vi "canDataSort.vi"() -> ()   [LabVIEW 2023] (continued)
    3823  0CF102A7   00000004    8        30\t75\tE0\t2E\t80\tFF\tFF\tFD\r\n      3823  0CF101A7   00000004    8        68\t00\t97\tCC\t00\t19\t39\tD9\r\n      3822  1FFFFFFF   00000004    8        00\t20\tFF\tFF\tFF\tFF\tFF\tFF\r\n      3812  1FFFFFFF   00000004    8        00\t00\tFF\tFF\tFF\tFF\tFF\tFF\r\n      3803  0CF102A7   00000004    8        30\t75\tE0\t2E\t80\tFF\tFF\tFD\r\n      3844  0CF103A7   00000004    8        17\t1F\t08\t60\tB1\t1F\t08\t5E\r\n      3844  0CF102A7   00000004    8        30\t75\tE0\t2E\t80\tFF\tFF\tFD\r\n      3843  0C3C4D4A   00000004    8        BE\tFF\tFF\t7F\t18\tFF\tFF\t5E\r\n      3843  0CF101A7   00000004    8        68\t00\t97\tCC\t00\t19\t39\tDA\r\n      3842  18F120F0   00000004    8        2B\t75\t60\tB1\tB0\t01\tFF\tFF\r\n      3841  18F11FF0   00000004    8        FF\t3F\t90\t68\t88\t1B\t10\tEC\r\n      3832  1FFFFFFF   00000004    8        00\t00\tFF\tFF\tFF\tFF\tFF\tFF\r\n      3823  0CF102A7   00000004    8        30\t75\tE0\t2E\t80\tFF\tFF\tFD\r\n      3823  0CF101A7   00000004    8        68\t00\t97\tCC\t00\t19\t39\tD9\r\n      3822  1FFFFFFF   00000004    8        00\t20\tFF\tFF\tFF\tFF\tFF\tFF\r\n      3812  1FFFFFFF   00000004    8        00\t00\tFF\tFF\tFF\tFF\tFF\tFF\r\n      3845  0CF104A7   00000004    8        F0\t60\t22\tFC\tFF\tFF\tFF\t5E\r\n      3844  0CF103A7   00000004    8        17\t1F\t08\t60\tB1\t1F\t08\t5E\r\n      3844  0CF102A7   00000004    8        30\t75\tE0\t2E\t80\tFF\tFF\tFD\r\n      3843  0C3C4D4A   00000004    8        BE\tFF\tFF\t7F\t18\tFF\tFF\t5E\r\n      3843  0CF101A7   00000004    8        68\t00\t97\tCC\t00\t19\t39\tDA\r\n      3842  18F120F0   00000004    8        2B\t75\t60\tB1\tB0\t01\tFF\tFF\r\n      3841  18F11FF0   00000004    8        FF\t3F\t90\t68\t88\t1B\t10\tEC\r\n      3832  1FFFFFFF   00000004    8        00\t00\tFF\tFF\tFF\tFF\tFF\tFF\r\n      3823  0CF102A7   00000004    8        30\t75\tE0\t2E\t80\tFF\tFF\tFD\r\n      3823  0CF101A7   00000004    8        68\t00\t97\tCC\t00\t19\t39\tD9\r\n      3822  1FFFFFFF   00000004    8        00\t20\tFF\tFF\tFF\tFF\tFF\tFF\r\n      3845  18F106A7   00000004    8        00\tF7\tFF\tFF\tFF\tFF\tFF\tBD\r\n      3845  0CF104A7   00000004    8        F0\t60\t22\tFC\tFF\tFF\tFF\t5E\r\n      3844  0CF103A7   00000004    8        17\t1F\t08\t60\tB1\t1F\t08\t5E\r\n      3844  0CF102A7   00000004    8        30\t75\tE0\t2E\t80\tFF\tFF\tFD\r\n      3843  0C3C4D4A   00000004    8        BE\tFF\tFF\t7F\t18\tFF\tFF\t5E\r\n      3843  0CF101A7   00000004    8        68\t00\t97\tCC\t00\t19\t39\tDA\r\n      3842  18F120F0   00000004    8        2B\t75\t60\tB1\tB0\t01\tFF\tFF\r\n      3841  18F11FF0   00000004    8        FF\t3F\t90\t68\t88\t1B\t10\tEC\r\n      3832  1FFFFFFF   00000004    8        00\t00\tFF\tFF\tFF\tFF\tFF\tFF\r\n      3823  0CF102A7   00000004    8        30\t75\tE0\t2E\t80\tFF\tFF\tFD\r\n      3823  0CF101A7   00000004    8        68\t00\t97\tCC\t00\t19\t39\tD9\r\n      3846  18F121F0   00000004    8        09\t33\t00\t00\tFF\tFF\tB0\t01\r\n      3845  18F106A7   00000004    8        00\tF7\tFF\tFF\tFF\tFF\tFF\tBD\r\n      3845  0CF104A7   00000004    8        F0\t60\t22\tFC\tFF\tFF\tFF\t5E\r\n      3844  0CF103A7   00000004    8        17\t1F\t08\t60\tB1\t1F\t08\t5E\r\n      3844  0CF102A7   00000004    8        30\t75\tE0\t2E\t80\tFF\tFF\tFD\r\n      3843  0C3C4D4A   00000004    8        BE\tFF\tFF\t7F\t18\tFF\tFF\t5E\r\n      3843  0CF101A7   00000004    8        68\t00\t97\tCC\t00\t19\t39\tDA\r\n      3842  18F120F0   00000004    8        2B\t75\t60\tB1\tB0\t01\tFF\tFF\r\n      3841  18F11FF0   00000004    8        FF\t3F\t90\t68\t88\t1B\t10\tEC\r\n      3832  1FFFFFFF   00000004    8        00\t00\tFF\tFF\tFF\tFF\tFF\tFF\r\n      3823  0CF102A7   00000004    8        30\t75\tE0\t2E\t80\tFF\tFF\tFD\r\n      3847  1FFFFFFF   00000004    8        00\t00\tFF\tFF\tFF\tFF\tFF\tFF\r\n      3846  18F121F0   00000004    8        09\t33\t00\t00\tFF\tFF\tB0\t01\r\n      3845  18F106A7   00000004    8        00\tF7\tFF\tFF\tFF\tFF\tFF\tBD\r\n      3845  0CF104A7   00000004    8        F0\t60\t22\tFC\tFF\tFF\tFF\t5E\r\n      3844  0CF103A7   00000004    8        17\t1F\t08\t60\tB1\t1F\t08\t5E\r\n      3844  0CF102A7   00000004    8        30\t75\tE0\t2E\t80\tFF\tFF\tFD\r\n      3843  0C3C4D4A   00000004    8        BE\tFF\tFF\t7F\t18\tFF\tFF\t5E\r\n      3843  0CF101A7   00000004    8        68\t00\t97\tCC\t00\t19\t39\tDA\r\n      3842  18F120F0   00000004    8        2B\t75\t60\tB1\tB0\t01\tFF\tFF\r\n      3841  18F11FF0   00000004    8        FF\t3F\t90\t68\t88\t1B\t10\tEC\r\n      3832  1FFFFFFF   00000004    8        00\t00\tFF\tFF\tFF\tFF\tFF\tFF\r\n      3852  1FFFFFFF   00000004    8        00\t00\tFF\tFF\tFF\tFF\tFF\tFF\r\n      3847  1FFFFFFF   00000004    8        00\t00\tFF\tFF\tFF\tFF\tFF\tFF\r\n      3846  18F121F0   00000004    8        09\t33\t00\t00\tFF\tFF\tB0\t01\r\n      3845  18F106A7   00000004    8        00\tF7\tFF\tFF\tFF\tFF\tFF\tBD\r\n      3845  0CF104A7   00000004    8        F0\t60\t22\tFC\tFF\tFF\tFF\t5E\r\n      3844  0CF103A7   00000004    8        17\t1F\t08\t60\tB1\t1F\t08\t5E\r\n      3844  0CF102A7   00000004    8        30\t75\tE0\t2E\t80\tFF\tFF\tFD\r\n      3843  0C3C4D4A   00000004    8        BE\tFF\tFF\t7F\t18\tFF\tFF\t5E\r\n      3843  0CF101A7   00000004    8        68\t00\t97\tCC\t00\t19\t39\tDA\r\n      3842  18F120F0   00000004    8        2B\t75\t60\tB1\tB0\t01\tFF\tFF\r\n      3841  18F11FF0   00000004    8        FF\t3F\t90\t68\t88\t1B\t10\tEC\r\n      3862  1FFFFFFF   00000004    8        00\t00\tFF\tFF\tFF\tFF\tFF\tFF\r\n      3852  1FFFFFFF   00000004    8        00\t00\tFF\tFF\tFF\tFF\tFF\tFF\r\n      3847  1FFFFFFF   00000004    8        00\t00\tFF\tFF\tFF\tFF\tFF\tFF\r\n      3846  18F121F0   00000004    8        09\t33\t00\t00\tFF\tFF\tB0\t01\r\n      3845  18F106A7   00000004    8        00\tF7\tFF\tFF\tFF\tFF\tFF\tBD\r\n      3845  0CF104A7   00000004    8        F0\t60\t22\tFC\tFF\tFF\tFF\t5E\r\n      3844  0CF103A7   00000004    8        17\t1F\t08\t60\tB1\t1F\t08\t5E\r\n      3844  0CF102A7   00000004    8        30\t75\tE0\t2E\t80\tFF\tFF\tFD\r\n      3843  0C3C4D4A   00000004    8        BE\tFF\tFF\t7F\t18\tFF\tFF\t5E\r\n      3843  0CF101A7   00000004    8        68\t00\t97\tCC\t00\t19\t39\tDA\r\n      3842  18F120F0   00000004    8        2B\t75\t60\tB1\tB0\t01\tFF\tFF\r\n      3863  0CF101A7   00000004    8        68\t00\t97\tCC\t00\t19\t39\tDB\r\n      3862  1FFFFFFF   00000004    8        00\t00\tFF\tFF\tFF\tFF\tFF\tFF\r\n      3852  1FFFFFFF   00000004    8        00\t00\tFF\tFF\tFF\tFF\tFF\tFF\r\n      3847  1FFFFFFF   00000004    8        00\t00\tFF\tFF\tFF\tFF\tFF\tFF\r\n      3846  18F121F0   00000004    8        09\t33\t00\t00\tFF\tFF\tB0\t01\r\n      3845  18F106A7   00000004    8        00\tF7\tFF\tFF\tFF\tFF\tFF\tBD\r\n      3845  0CF104A7   00000004    8        F0\t60\t22\tFC\tFF\tFF\tFF\t5E\r\n      3844  0CF103A7   00000004    8        17\t1F\t08\t60\tB1\t1F\t08\t5E\r\n      3844  0CF102A7   00000004    8        30\t75\tE0\t2E\t80\tFF\tFF\tFD\r\n      3843  0C3C4D4A   00000004    8        BE\tFF\tFF\t7F\t18\tFF\tFF\t5E\r\n      3843  0CF101A7   00000004    8        68\t00\t97\tCC\t00\t19\t39\tDA\r\n      3863  0CF102A7   00000004    8        30\t75\tE0\t2E\t80\tFF\tFF\tFD\r\n      3863  0CF101A7   00000004    8        68\t00\t97\tCC\t00\t19\t39\tDB\r\n      3862  1FFFFFFF   00000004    8        00\t00\tFF\tFF\tFF\tFF\tFF\tFF\r\n      3852  1FFFFFFF   00000004    8        00\t00\tFF\tFF\tFF\tFF\tFF\tFF\r\n      3847  1FFFFFFF   00000004    8        00\t00\tFF\tFF\tFF\tFF\tFF\tFF\r\n      3846  18F121F0   00000004    8        09\t33\t00\t00\tFF\tFF\tB0\t01\r\n      3845  18F106A7   00000004    8        00\tF7\tFF\tFF\tFF\tFF\tFF\tBD\r\n      3845  0CF104A7   00000004    8        F0\t60\t22\tFC\tFF\tFF\tFF\t5E\r\n      3844  0CF103A7   00000004    8        17\t1F\t08\t60\tB1\t1F\t08\t5E\r\n      3844  0CF102A7   00000004    8        30\t75\tE0\t2E\t80\tFF\tFF\tFD\r\n      3843  0C3C4D4A   00000004    8        BE\tFF\tFF\t7F\t18\tFF\tFF\t5E\r\n      3872  1FFFFFFF   00000004    8        00\t00\tFF\tFF\tFF\tFF\tFF\tFF\r\n      3863  0CF102A7   00000004    8        30\t75\tE0\t2E\t80\tFF\tFF\tFD\r\n      3863  0CF101A7   00000004    8        68\t00\t97\tCC\t00\t19\t39\tDB\r\n      3862  1FFFFFFF   00000004    8        00\t00\tFF\tFF\tFF\tFF\tFF\tFF\r\n      3852  1FFFFFFF   00000004    8        00\t00\tFF\tFF\tFF\tFF\tFF\tFF\r\n      3847  1FFFFFFF   00000004    8        00\t00\tFF\tFF\tFF\tFF\tFF\tFF\r\n      3846  18F121F0   00000004    8        09\t33\t00\t00\tFF\tFF\tB0\t01\r\n      3845  18F106A7   00000004    8        00\tF7\tFF\tFF\tFF\tFF\tFF\tBD\r\n      3845  0CF104A7   00000004    8        F0\t60\t22\tFC\tFF\tFF\tFF\t5E\r\n      3844  0CF103A7   00000004    8        17\t1F\t08\t60\tB1\t1F\t08\t5E\r\n      3844  0CF102A7   00000004    8        30\t75\tE0\t2E\t80\tFF\tFF\tFD\r\n      3882  1FFFFFFF   00000004    8        00\t00\tFF\tFF\tFF\tFF\tFF\tFF\r\n      3872  1FFFFFFF   00000004    8        00\t00\tFF\tFF\tFF\tFF\tFF\tFF\r\n      3863  0CF102A7   00000004    8        30\t75\tE0\t2E\t80\tFF\tFF\tFD\r\n      3863  0CF101A7   00000004    8        68\t00\t97\tCC\t00\t19\t39\tDB\r\n      3862  1FFFFFFF   00000004    8        00\t00\tFF\tFF\tFF\tFF\tFF\tFF\r\n      3852  1FFFFFFF   00000004    8        00\t00\tFF\tFF\tFF\tFF\tFF\tFF\r\n      3847  1FFFFFFF   00000004    8        00\t00\tFF\tFF\tFF\tFF\tFF\tFF\r\n      3846  18F121F0   00000004    8        09\t33\t00\t00\tFF\tFF\tB0\t01\r\n      3845  18F106A7   00000004    8        00\tF7\tFF\tFF\tFF\tFF\tFF\tBD\r\n      3845  0CF104A7   00000004    8        F0\t60\t22\tFC\tFF\tFF\tFF\t5E\r\n      3844  0CF103A7   00000004    8        17\t1F\t08\t60\tB1\t1F\t08\t5E\r\n      3883  0CF101A7   00000004    8        68\t00\t97\tCC\t00\t19\t39\tDC\r\n      3882  1FFFFFFF   00000004    8        00\t00\tFF\tFF\tFF\tFF\tFF\tFF\r\n      3872  1FFFFFFF   00000004    8        00\t00\tFF\tFF\tFF\tFF\tFF\tFF\r\n      3863  0CF102A7   00000004    8        30\t75\tE0\t2E\t80\tFF\tFF\tFD\r\n      3863  0CF101A7   00000004    8        68\t00\t97\tCC\t00\t19\t39\tDB\r\n      3862  1FFFFFFF   00000004    8        00\t00\tFF\tFF\tFF\tFF\tFF\tFF\r\n      3852  1FFFFFFF   00000004    8        00\t00\tFF\tFF\tFF\tFF\tFF\tFF\r\n      3847  1FFFFFFF   00000004    8        00\t00\tFF\tFF\tFF\tFF\tFF\tFF\r\n      3846  18F121F0   00000004    8        09\t33\t00\t00\tFF\tFF\tB0\t01\r\n      3845  18F106A7   00000004    8        00\tF7\tFF\tFF\tFF\tFF\tFF\tBD\r\n      3845  0CF104A7   00000004    8        F0\t60\t22\tFC\tFF\tFF\tFF\t5E\r\n      3883  0CF102A7   00000004    8        30\t75\tE0\t2E\t80\tFF\tFF\tFD\r\n      3883  0CF101A7   00000004    8        68\t00\t97\tCC\t00\t19\t39\tDC\r\n      3882  1FFFFFFF   00000004    8        00\t00\tFF\tFF\tFF\tFF\tFF\tFF\r\n      3872  1FFFFFFF   00000004    8        00\t00\tFF\tFF\tFF\tFF\tFF\tFF\r\n      3863  0CF102A7   00000004    8        30\t75\tE0\t2E\t80\tFF\tFF\tFD\r\n      3863  0CF101A7   00000004    8        68\t00\t97\tCC\t00\t19\t39\tDB\r\n      3862  1FFFFFFF   00000004    8        00\t00\tFF\tFF\tFF\tFF\tFF\tFF\r\n      3852  1FFFFFFF   00000004    8        00\t00\tFF\tFF\tFF\tFF\tFF\tFF\r\n      3847  1FFFFFFF   00000004    8        00\t00\tFF\tFF\tFF\tFF\tFF\tFF\r\n      3846  18F121F0   00000004    8        09\t33\t00\t00\tFF\tFF\tB0\t01\r\n      3845  18F106A7   00000004    8        00\tF7\tFF\tFF\tFF\tFF\tFF\tBD\r\n      3892  1FFFFFFF   00000004    8        00\t00\tFF\tFF\tFF\tFF\tFF\tFF\r\n      3883  0CF102A7   00000004    8        30\t75\tE0\t2E\t80\tFF\tFF\tFD\r\n      3883  0CF101A7   00000004    8        68\t00\t97\tCC\t00\t19\t39\tDC\r\n      3882  1FFFFFFF   00000004    8        00\t00\tFF\tFF\tFF\tFF\tFF\tFF\r\n      3872  1FFFFFFF   00000004    8        00\t00\tFF\tFF\tFF\tFF\tFF\tFF\r\n      3863  0CF102A7   00000004    8        30\t75\tE0\t2E\t80\tFF\tFF\tFD\r\n      3863  0CF101A7   00000004    8        68\t00\t97\tCC\t00\t19\t39\tDB\r\n      3862  1FFFFFFF   00000004    8        00\t00\tFF\tFF\tFF\tFF\tFF\tFF\r\n      3852  1FFFFFFF   00000004    8        00\t00\tFF\tFF\tFF\tFF\tFF\tFF\r\n      3847  1FFFFFFF   00000004    8        00\t00\tFF\tFF\tFF\tFF\tFF\tFF\r\n      3846  18F121F0   00000004    8        09\t33\t00\t00\tFF\tFF\tB0\t01\r\n      3893  18F106A7   00000004    8        00\tF7\tFF\tFF\tFF\tFF\tFF\tBE\r\n      3892  1FFFFFFF   00000004    8        00\t00\tFF\tFF\tFF\tFF\tFF\tFF\r\n      3883  0CF102A7   00000004    8        30\t75\tE0\t2E\t80\tFF\tFF\tFD\r\n      3883  0CF101A7   00000004    8        68\t00\t97\tCC\t00\t19\t39\tDC\r\n      3882  1FFFFFFF   00000004    8        00\t00\tFF\tFF\tFF\tFF\tFF\tFF\r\n      3872  1FFFFFFF   00000004    8        00\t00\tFF\tFF\tFF\tFF\tFF\tFF\r\n      3863  0CF102A7   00000004    8        30\t75\tE0\t2E\t80\tFF\tFF\tFD\r\n      3863  0CF101A7   00000004    8        68\t00\t97\tCC\t00\t19\t39\tDB\r\n      3862  1FFFFFFF   00000004    8        00\t00\tFF\tFF\tFF\tFF\tFF\tFF\r\n      3852  1FFFFFFF   00000004    8        00\t00\tFF\tFF\tFF\tFF\tFF\tFF\r\n      3847  1FFFFFFF   00000004    8        00\t00\tFF\tFF\tFF\tFF\tFF\tFF\r\n      3902  1FFFFFFF   00000004    8        00\t20\tFF\tFF\tFF\tFF\tFF\tFF\r\n      3893  18F106A7   00000004    8        00\tF7\tFF\tFF\tFF\tFF\tFF\tBE\r\n      3892  1FFFFFFF   00000004    8        00\t00\tFF\tFF\tFF\tFF\tFF\tFF\r\n      3883  0CF102A7   00000004    8        30\t75\tE0\t2E\t80\tFF\tFF\tFD\r\n      3883  0CF101A7   00000004    8        68\t00\t97\tCC\t00\t19\t39\tDC\r\n      3882  1FFFFFFF   00000004    8        00\t00\tFF\tFF\tFF\tFF\tFF\tFF\r\n      3872  1FFFFFFF   00000004    8        00\t00\tFF\tFF\tFF\tFF\tFF\tFF\r\n      3863  0CF102A7   00000004    8        30\t75\tE0\t2E\t80\tFF\tFF\tFD\r\n      3863  0CF101A7   00000004    8        68\t00\t97\tCC\t00\t19\t39\tDB\r\n      3862  1FFFFFFF   00000004    8        00\t00\tFF\tFF\tFF\tFF\tFF\tFF\r\n      3852  1FFFFFFF   00000004    8        00\t00\tFF\tFF\tFF\tFF\tFF\tFF\r\n      3902  0CF101A7   00000004    8        68\t00\t97\tCC\t00\t19\t39\tDD\r\n      3902  1FFFFFFF   00000004    8        00\t20\tFF\tFF\tFF\tFF\tFF\tFF\r\n      3893  18F106A7   00000004    8        00\tF7\tFF\tFF\tFF\tFF\tFF\tBE\r\n      3892  1FFFFFFF   00000004    8        00\t00\tFF\tFF\tFF\tFF\tFF\tFF\r\n      3883  0CF102A7   00000004    8        30\t75\tE0\t2E\t80\tFF\tFF\tFD\r\n      3883  0CF101A7   00000004    8        68\t00\t97\tCC\t00\t19\t39\tDC\r\n      3882  1FFFFFFF   00000004    8        00\t00\tFF\tFF\tFF\tFF\tFF\tFF\r\n      3872  1FFFFFFF   00000004    8        00\t00\tFF\tFF\tFF\tFF\tFF\tFF\r\n      3863  0CF102A7   00000004    8        30\t75\tE0\t2E\t80\tFF\tFF\tFD\r\n      3863  0CF101A7   00000004    8        68\t00\t97\tCC\t00\t19\t39\tDB\r\n      3862  1FFFFFFF   00000004    8        00\t00\tFF\tFF\tFF\tFF\tFF\tFF\r\n      3903  0CF102A7   00000004    8        30\t75\tE0\t2E\t80\tFF\tFF\tFD\r\n      3902  0CF101A7   00000004    8        68\t00\t97\tCC\t00\t19\t39\tDD\r\n      3902  1FFFFFFF   00000004    8        00\t20\tFF\tFF\tFF\tFF\tFF\tFF\r\n      3893  18F106A7   00000004    8        00\tF7\tFF\tFF\tFF\tFF\tFF\tBE\r\n      3892  1FFFFFFF   00000004    8        00\t00\tFF\tFF\tFF\tFF\tFF\tFF\r\n      3883  0CF102A7   00000004    8        30\t75\tE0\t2E\t80\tFF\tFF\tFD\r\n      3883  0CF101A7   00000004    8        68\t00\t97\tCC\t00\t19\t39\tDC\r\n      3882  1FFFFFFF   00000004    8        00\t00\tFF\tFF\tFF\tFF\tFF\tFF\r\n      3872  1FFFFFFF   00000004    8        00\t00\tFF\tFF\tFF\tFF\tFF\tFF\r\n      3863  0CF102A7   00000004    8        30\t75\tE0\t2E\t80\tFF\tFF\tFD\r\n      3863  0CF101A7   00000004    8        68\t00\t97\tCC\t00\t19\t39\tDB\r\n      3912  1FFFFFFF   00000004    8        00\t00\tFF\tFF\tFF\tFF\tFF\tFF\r\n      3903  0CF102A7   00000004    8        30\t75\tE0\t2E\t80\tFF\tFF\tFD\r\n      3902  0CF101A7   00000004    8        68\t00\t97\tCC\t00\t19\t39\tDD\r\n      3902  1FFFFFFF   00000004    8        00\t20\tFF\tFF\tFF\tFF\tFF\tFF\r\n      3893  18F106A7   00000004    8        00\tF7\tFF\tFF\tFF\tFF\tFF\tBE\r\n      3892  1FFFFFFF   00000004    8        00\t00\tFF\tFF\tFF\tFF\tFF\tFF\r\n      3883  0CF102A7   00000004    8        30\t75\tE0\t2E\t80\tFF\tFF\tFD\r\n      3883  0CF101A7   00000004    8        68\t00\t97\tCC\t00\t19\t39\tDC\r\n      3882  1FFFFFFF   00000004    8        00\t00\tFF\tFF\tFF\tFF\tFF\tFF\r\n      3872  1FFFFFFF   00000004    8        00\t00\tFF\tFF\tFF\tFF\tFF\tFF\r\n      3863  0CF102A7   00000004    8        30\t75\tE0\t2E\t80\tFF\tFF\tFD\r\n      3922  1FFFFFFF   00000004    8        00\t00\tFF\tFF\tFF\tFF\tFF\tFF\r\n      3912  1FFFFFFF   00000004    8        00\t00\tFF\tFF\tFF\tFF\tFF\tFF\r\n      3903  0CF102A7   00000004    8        30\t75\tE0\t2E\t80\tFF\tFF\tFD\r\n      3902  0CF101A7   00000004    8        68\t00\t97\tCC\t00\t19\t39\tDD\r\n      3902  1FFFFFFF   00000004    8        00\t20\tFF\tFF\tFF\tFF\tFF\tFF\r\n      3893  18F106A7   00000004    8        00\tF7\tFF\tFF\tFF\tFF\tFF\tBE\r\n      3892  1FFFFFFF   00000004    8        00\t00\tFF\tFF\tFF\tFF\tFF\tFF\r\n      3883  0CF102A7   00000004    8        30\t75\tE0\t2E\t80\tFF\tFF\tFD\r\n      3883  0CF101A7   00000004    8        68\t00\t97\tCC\t00\t19\t39\tDC\r\n      3882  1FFFFFFF   00000004    8        00\t00\tFF\tFF\tFF\tFF\tFF\tFF\r\n      3872  1FFFFFFF   00000004    8        00\t00\tFF\tFF\tFF\tFF\tFF\tFF\r\n      3923  0CF101A7   00000004    8        68\t00\t97\tCC\t00\t19\t39\tDE\r\n      3922  1FFFFFFF   00000004    8        00\t00\tFF\tFF\tFF\tFF\tFF\tFF\r\n      3912  1FFFFFFF   00000004    8        00\t00\tFF\tFF\tFF\tFF\tFF\tFF\r\n      3903  0CF102A7   00000004    8        30\t75\tE0\t2E\t80\tFF\tFF\tFD\r\n      3902  0CF101A7   00000004    8        68\t00\t97\tCC\t00\t19\t39\tDD\r\n      3902  1FFFFFFF   00000004    8        00\t20\tFF\tFF\tFF\tFF\tFF\tFF\r\n      3893  18F106A7   00000004    8        00\tF7\tFF\tFF\tFF\tFF\tFF\tBE\r\n      3892  1FFFFFFF   00000004    8        00\t00\tFF\tFF\tFF\tFF\tFF\tFF\r\n      3883  0CF102A7   00000004    8        30\t75\tE0\t2E\t80\tFF\tFF\tFD\r\n      3883  0CF101A7   00000004    8        68\t00\t97\tCC\t00\t19\t39\tDC\r\n      3882  1FFFFFFF   00000004    8        00\t00\tFF\tFF\tFF\tFF\tFF\tFF\r\n      3923  0CF102A7   00000004    8        30\t75\tE0\t2E\t80\tFF\tFF\tFD\r\n      3923  0CF101A7   00000004    8        68\t00\t97\tCC\t00\t19\t39\tDE\r\n      3922  1FFFFFFF   00000004    8        00\t00\tFF\tFF\tFF\tFF\tFF\tFF\r\n      3912  1FFFFFFF   00000004    8        00\t00\tFF\tFF\tFF\tFF\tFF\tFF\r\n      3903  0CF102A7   00000004    8        30\t75\tE0\t2E\t80\tFF\tFF\tFD\r\n      3902  0CF101A7   00000004    8        68\t00\t97\tCC\t00\t19\t39\tDD\r\n      3902  1FFFFFFF   00000004    8        00\t20\tFF\tFF\tFF\tFF\tFF\tFF\r\n      3893  18F106A7   00000004    8        00\tF7\tFF\tFF\tFF\tFF\tFF\tBE\r\n      3892  1FFFFFFF   00000004    8        00\t00\tFF\tFF\tFF\tFF\tFF\tFF\r\n      3883  0CF102A7   00000004    8        30\t75\tE0\t2E\t80\tFF\tFF\tFD\r\n      3883  0CF101A7   00000004    8        68\t00\t97\tCC\t00\t19\t39\tDC\r\n      3932  1FFFFFFF   00000004    8        00\t00\tFF\tFF\tFF\tFF\tFF\tFF\r\n      3923  0CF102A7   00000004    8        30\t75\tE0\t2E\t80\tFF\tFF\tFD\r\n      3923  0CF101A7   00000004    8        68\t00\t97\tCC\t00\t19\t39\tDE\r\n      3922  1FFFFFFF   00000004    8        00\t00\tFF\tFF\tFF\tFF\tFF\tFF\r\n      3912  1FFFFFFF   00000004    8        00\t00\tFF\tFF\tFF\tFF\tFF\tFF\r\n      3903  0CF102A7   00000004    8        30\t75\tE0\t2E\t80\tFF\tFF\tFD\r\n      3902  0CF101A7   00000004    8        68\t00\t97\tCC\t00\t19\t39\tDD\r\n      3902  1FFFFFFF   00000004    8        00\t20\tFF\tFF\tFF\tFF\tFF\tFF\r\n      3893  18F106A7   00000004    8        00\tF7\tFF\tFF\tFF\tFF\tFF\tBE\r\n      3892  1FFFFFFF   00000004    8        00\t00\tFF\tFF\tFF\tFF\tFF\tFF\r\n      3883  0CF102A7   00000004    8        30\t75\tE0\t2E\t80\tFF\tFF\tFD\r\n      3941  18F11FF0   00000004    8        FF\t3F\t90\t68\t88\t1B\t10\tFC\r\n      3932  1FFFFFFF   00000004    8        00\t00\tFF\tFF\tFF\tFF\tFF\tFF\r\n      3923  0CF102A7   00000004    8        30\t75\tE0\t2E\t80\tFF\tFF\tFD\r\n      3923  0CF101A7   00000004    8        68\t00\t97\tCC\t00\t19\t39\tDE\r\n      3922  1FFFFFFF   00000004    8        00\t00\tFF\tFF\tFF\tFF\tFF\tFF\r\n      3912  1FFFFFFF   00000004    8        00\t00\tFF\tFF\tFF\tFF\tFF\tFF\r\n      3903  0CF102A7   00000004    8        30\t75\tE0\t2E\t80\tFF\tFF\tFD\r\n      3902  0CF101A7   00000004    8        68\t00\t97\tCC\t00\t19\t39\tDD\r\n      3902  1FFFFFFF   00000004    8        00\t20\tFF\tFF\tFF\tFF\tFF\tFF\r\n      3893  18F106A7   00000004    8        00\tF7\tFF\tFF\tFF\tFF\tFF\tBE\r\n      3892  1FFFFFFF   00000004    8        00\t00\tFF\tFF\tFF\tFF\tFF\tFF\r\n      3942  18F120F0   00000004    8        2B\t75\t60\tB1\tB0\t01\tFF\tFF\r\n      3941  18F11FF0   00000004    8        FF\t3F\t90\t68\t88\t1B\t10\tFC\r\n      3932  1FFFFFFF   00000004    8        00\t00\tFF\tFF\tFF\tFF\tFF\tFF\r\n      3923  0CF102A7   00000004    8        30\t75\tE0\t2E\t80\tFF\tFF\tFD\r\n      3923  0CF101A7   00000004    8        68\t00\t97\tCC\t00\t19\t39\tDE\r\n      3922  1FFFFFFF   00000004    8        00\t00\tFF\tFF\tFF\tFF\tFF\tFF\r\n      3912  1FFFFFFF   00000004    8        00\t00\tFF\tFF\tFF\tFF\tFF\tFF\r\n      3903  0CF102A7   00000004    8        30\t75\tE0\t2E\t80\tFF\tFF\tFD\r\n      3902  0CF101A7   00000004    8        68\t00\t97\tCC\t00\t19\t39\tDD\r\n      3902  1FFFFFFF   00000004    8        00\t20\tFF\tFF\tFF\tFF\tFF\tFF\r\n      3893  18F106A7   00000004    8        00\tF7\tFF\tFF\tFF\tFF\tFF\tBE\r\n      3943  0CF101A7   00000004    8        68\t00\t97\tCC\t00\t19\t39\tDF\r\n      3942  18F120F0   00000004    8        2B\t75\t60\tB1\tB0\t01\tFF\tFF\r\n      3941  18F11FF0   00000004    8        FF\t3F\t90\t68\t88\t1B\t10\tFC\r\n      3932  1FFFFFFF   00000004    8        00\t00\tFF\tFF\tFF\tFF\tFF\tFF\r\n      3923  0CF102A7   00000004    8        30\t75\tE0\t2E\t80\tFF\tFF\tFD\r\n      3923  0CF101A7   00000004    8        68\t00\t97\tCC\t00\t19\t39\tDE\r\n      3922  1FFFFFFF   00000004    8        00\t00\tFF\tFF\tFF\tFF\tFF\tFF\r\n      3912  1FFFFFFF   00000004    8        00\t00\tFF\tFF\tFF\tFF\tFF\tFF\r\n      3903  0CF102A7   00000004    8        30\t75\tE0\t2E\t80\tFF\tFF\tFD\r\n      3902  0CF101A7   00000004    8        68\t00\t97\tCC\t00\t19\t39\tDD\r\n      3902  1FFFFFFF   00000004    8        00\t20\tFF\tFF\tFF\tFF\tFF\tFF\r\n      3943  0C3C4D4A   00000004    8        BE\tFF\tFF\t7F\t18\tFF\tFF\t5F\r\n      3943  0CF101A7   00000004    8        68\t00\t97\tCC\t00\t19\t39\tDF\r\n      3942  18F120F0   00000004    8        2B\t75\t60\tB1\tB0\t01\tFF\tFF\r\n      3941  18F11FF0   00000004    8        FF\t3F\t90\t68\t88\t1B\t10\tFC\r\n      3932  1FFFFFFF   00000004    8        00\t00\tFF\tFF\tFF\tFF\tFF\tFF\r\n      3923  0CF102A7   00000004    8        30\t75\tE0\t2E\t80\tFF\tFF\tFD\r\n      3923  0CF101A7   00000004    8        68\t00\t97\tCC\t00\t19\t39\tDE\r\n      3922  1FFFFFFF   00000004    8        00\t00\tFF\tFF\tFF\tFF\tFF\tFF\r\n      3912  1FFFFFFF   00000004    8        00\t00\tFF\tFF\tFF\tFF\tFF\tFF\r\n      3903  0CF102A7   00000004    8        30\t75\tE0\t2E\t80\tFF\tFF\tFD\r\n      3902  0CF101A7   00000004    8        68\t00\t97\tCC\t00\t19\t39\tDD\r\n      3944  0CF102A7   00000004    8        30\t75\tE0\t2E\t80\tFF\tFF\tFD\r\n      3943  0C3C4D4A   00000004    8        BE\tFF\tFF\t7F\t18\tFF\tFF\t5F\r\n      3943  0CF101A7   00000004    8        68\t00\t97\tCC\t00\t19\t39\tDF\r\n      3942  18F120F0   00000004    8        2B\t75\t60\tB1\tB0\t01\tFF\tFF\r\n      3941  18F11FF0   00000004    8        FF\t3F\t90\t68\t88\t1B\t10\tFC\r\n      3932  1FFFFFFF   00000004    8        00\t00\tFF\tFF\tFF\tFF\tFF\tFF\r\n      3923  0CF102A7   00000004    8        30\t75\tE0\t2E\t80\tFF\tFF\tFD\r\n      3923  0CF101A7   00000004    8        68\t00\t97\tCC\t00\t19\t39\tDE\r\n      3922  1FFFFFFF   00000004    8        00\t00\tFF\tFF\tFF\tFF\tFF\tFF\r\n      3912  1FFFFFFF   00000004    8        00\t00\tFF\tFF\tFF\tFF\tFF\tFF\r\n      3903  0CF102A7   00000004    8        30\t75\tE0\t2E\t80\tFF\tFF\tFD\r\n      3944  0CF103A7   00000004    8        17\t1F\t08\t60\tB1\t1F\t08\t5F\r\n      3944  0CF102A7   00000004    8        30\t75\tE0\t2E\t80\tFF\tFF\tFD\r\n      3943  0C3C4D4A   00000004    8        BE\tFF\tFF\t7F\t18\tFF\tFF\t5F\r\n      3943  0CF101A7   00000004    8        68\t00\t97\tCC\t00\t19\t39\tDF\r\n      3942  18F120F0   00000004    8        2B\t75\t60\tB1\tB0\t01\tFF\tFF\r\n      3941  18F11FF0   00000004    8        FF\t3F\t90\t68\t88\t1B\t10\tFC\r\n      3932  1FFFFFFF   00000004    8        00\t00\tFF\tFF\tFF\tFF\tFF\tFF\r\n      3923  0CF102A7   00000004    8        30\t75\tE0\t2E\t80\tFF\tFF\tFD\r\n      3923  0CF101A7   00000004    8        68\t00\t97\tCC\t00\t19\t39\tDE\r\n      3922  1FFFFFFF   00000004    8        00\t00\tFF\tFF\tFF\tFF\tFF\tFF\r\n      3912  1FFFFFFF   00000004    8        00\t00\tFF\tFF\tFF\tFF\tFF\tFF\r\n      3945  0CF104A7   00000004    8        F0\t60\t22\tFC\tFF\tFF\tFF\t5F\r\n      3944  0CF103A7   00000004    8        17\t1F\t08\t60\tB1\t1F\t08\t5F\r\n      3944  0CF102A7   00000004    8        30\t75\tE0\t2E\t80\tFF\tFF\tFD\r\n      3943  0C3C4D4A   00000004    8        BE\tFF\tFF\t7F\t18\tFF\tFF\t5F\r\n      3943  0CF101A7   00000004    8        68\t00\t97\tCC\t00\t19\t39\tDF\r\n      3942  18F120F0   00000004    8        2B\t75\t60\tB1\tB0\t01\tFF\tFF\r\n      3941  18F11FF0   00000004    8        FF\t3F\t90\t68\t88\t1B\t10\tFC\r\n      3932  1FFFFFFF   00000004    8        00\t00\tFF\tFF\tFF\tFF\tFF\tFF\r\n      3923  0CF102A7   00000004    8        30\t75\tE0\t2E\t80\tFF\tFF\tFD\r\n      3923  0CF101A7   00000004    8        68\t00\t97\tCC\t00\t19\t39\tDE\r\n      3922  1FFFFFFF   00000004    8        00\t00\tFF\tFF\tFF\tFF\tFF\tFF\r\n      3945  18F106A7   00000004    8        00\tF7\tFF\tFF\tFF\tFF\tFF\tBF\r\n      3945  0CF104A7   00000004    8        F0\t60\t22\tFC\tFF\tFF\tFF\t5F\r\n      3944  0CF103A7   00000004    8        17\t1F\t08\t60\tB1\t1F\t08\t5F\r\n      3944  0CF102A7   00000004    8        30\t75\tE0\t2E\t80\tFF\tFF\tFD\r\n      3943  0C3C4D4A   00000004    8        BE\tFF\tFF\t7F\t18\tFF\tFF\t5F\r\n      3943  0CF101A7   00000004    8        68\t00\t97\tCC\t00\t19\t39\tDF\r\n      3942  18F120F0   00000004    8        2B\t75\t60\tB1\tB0\t01\tFF\tFF\r\n      3941  18F11FF0   00000004    8        FF\t3F\t90\t68\t88\t1B\t10\tFC\r\n      3932  1FFFFFFF   00000004    8        00\t00\tFF\tFF\tFF\tFF\tFF\tFF\r\n      3923  0CF102A7   00000004    8        30\t75\tE0\t2E\t80\tFF\tFF\tFD\r\n      3923  0CF101A7   00000004    8        68\t00\t97\tCC\t00\t19\t39\tDE\r\n      3946  18F121F0   00000004    8        09\t33\t00\t00\tFF\tFF\tB0\t01\r\n      3945  18F106A7   00000004    8        00\tF7\tFF\tFF\tFF\tFF\tFF\tBF\r\n      3945  0CF104A7   00000004    8        F0\t60\t22\tFC\tFF\tFF\tFF\t5F\r\n      3944  0CF103A7   00000004    8        17\t1F\t08\t60\tB1\t1F\t08\t5F\r\n      3944  0CF102A7   00000004    8        30\t75\tE0\t2E\t80\tFF\tFF\tFD\r\n      3943  0C3C4D4A   00000004    8        BE\tFF\tFF\t7F\t18\tFF\tFF\t5F\r\n      3943  0CF101A7   00000004    8        68\t00\t97\tCC\t00\t19\t39\tDF\r\n      3942  18F120F0   00000004    8        2B\t75\t60\tB1\tB0\t01\tFF\tFF\r\n      3941  18F11FF0   00000004    8        FF\t3F\t90\t68\t88\t1B\t10\tFC\r\n      3932  1FFFFFFF   00000004    8        00\t00\tFF\tFF\tFF\tFF\tFF\tFF\r\n      3923  0CF102A7   00000004    8        30\t75\tE0\t2E\t80\tFF\tFF\tFD\r\n      3947  1FFFFFFF   00000004    8        00\t00\tFF\tFF\tFF\tFF\tFF\tFF\r\n      3946  18F121F0   00000004    8        09\t33\t00\t00\tFF\tFF\tB0\t01\r\n      3945  18F106A7   00000004    8        00\tF7\tFF\tFF\tFF\tFF\tFF\tBF\r\n      3945  0CF104A7   00000004    8        F0\t60\t22\tFC\tFF\tFF\tFF\t5F\r\n      3944  0CF103A7   00000004    8        17\t1F\t08\t60\tB1\t1F\t08\t5F\r\n      3944  0CF102A7   00000004    8        30\t75\tE0\t2E\t80\tFF\tFF\tFD\r\n      3943  0C3C4D4A   00000004    8        BE\tFF\tFF\t7F\t18\tFF\tFF\t5F\r\n      3943  0CF101A7   00000004    8        68\t00\t97\tCC\t00\t19\t39\tDF\r\n      3942  18F120F0   00000004    8        2B\t75\t60\tB1\tB0\t01\tFF\tFF\r\n      3941  18F11FF0   00000004    8        FF\t3F\t90\t68\t88\t1B\t10\tFC\r\n      3932  1FFFFFFF   00000004    8        00\t00\tFF\tFF\tFF\tFF\tFF\tFF\r\n      3952  1FFFFFFF   00000004    8        00\t00\tFF\tFF\tFF\tFF\tFF\tFF\r\n      3947  1FFFFFFF   00000004    8        00\t00\tFF\tFF\tFF\tFF\tFF\tFF\r\n      3946  18F121F0   00000004    8        09\t33\t00\t00\tFF\tFF\tB0\t01\r\n      3945  18F106A7   00000004    8        00\tF7\tFF\tFF\tFF\tFF\tFF\tBF\r\n      3945  0CF104A7   00000004    8        F0\t60\t22\tFC\tFF\tFF\tFF\t5F\r\n      3944  0CF103A7   00000004    8        17\t1F\t08\t60\tB1\t1F\t08\t5F\r\n      3944  0CF102A7   00000004    8        30\t75\tE0\t2E\t80\tFF\tFF\tFD\r\n      3943  0C3C4D4A   00000004    8        BE\tFF\tFF\t7F\t18\tFF\tFF\t5F\r\n      3943  0CF101A7   00000004    8        68\t00\t97\tCC\t00\t19\t39\tDF\r\n      3942  18F120F0   00000004    8        2B\t75\t60\tB1\tB0\t01\tFF\tFF\r\n      3941  18F11FF0   00000004    8        FF\t3F\t90\t68\t88\t1B\t10\tFC\r\n      3962  1FFFFFFF   00000004    8        00\t00\tFF\tFF\tFF\tFF\tFF\tFF\r\n      3952  1FFFFFFF   00000004    8        00\t00\tFF\tFF\tFF\tFF\tFF\tFF\r\n      3947  1FFFFFFF   00000004    8        00\t00\tFF\tFF\tFF\tFF\tFF\tFF\r\n      3946  18F121F0   00000004    8        09\t33\t00\t00\tFF\tFF\tB0\t01\r\n      3945  18F106A7   00000004    8        00\tF7\tFF\tFF\tFF\tFF\tFF\tBF\r\n      3945  0CF104A7   00000004    8        F0\t60\t22\tFC\tFF\tFF\tFF\t5F\r\n      3944  0CF103A7   00000004    8        17\t1F\t08\t60\tB1\t1F\t08\t5F\r\n      3944  0CF102A7   00000004    8        30\t75\tE0\t2E\t80\tFF\tFF\tFD\r\n      3943  0C3C4D4A   00000004    8        BE\tFF\tFF\t7F\t18\tFF\tFF\t5F\r\n      3943  0CF101A7   00000004    8        68\t00\t97\tCC\t00\t19\t39\tDF\r\n      3942  18F120F0   00000004    8        2B\t75\t60\tB1\tB0\t01\tFF\tFF\r\n      3963  0CF101A7   00000004    8        68\t00\t97\tCC\t00\t19\t39\tE0\r\n      3962  1FFFFFFF   00000004    8        00\t00\tFF\tFF\tFF\tFF\tFF\tFF\r\n      3952  1FFFFFFF   00000004    8        00\t00\tFF\tFF\tFF\tFF\tFF\tFF\r\n      3947  1FFFFFFF   00000004    8        00\t00\tFF\tFF\tFF\tFF\tFF\tFF\r\n      3946  18F121F0   00000004    8        09\t33\t00\t00\tFF\tFF\tB0\t01\r\n      3945  18F106A7   00000004    8        00\tF7\tFF\tFF\tFF\tFF\tFF\tBF\r\n      3945  0CF104A7   00000004    8        F0\t60\t22\tFC\tFF\tFF\tFF\t5F\r\n      3944  0CF103A7   00000004    8        17\t1F\t08\t60\tB1\t1F\t08\t5F\r\n      3944  0CF102A7   00000004    8        30\t75\tE0\t2E\t80\tFF\tFF\tFD\r\n      3943  0C3C4D4A   00000004    8        BE\tFF\tFF\t7F\t18\tFF\tFF\t5F\r\n      3943  0CF101A7   00000004    8        68\t00\t97\tCC\t00\t19\t39\tDF\r\n      3963  0CF102A7   00000004    8        30\t75\tE0\t2E\t80\tFF\tFF\tFD\r\n      3963  0CF101A7   00000004    8        68\t00\t97\tCC\t00\t19\t39\tE0\r\n      3962  1FFFFFFF   00000004    8        00\t00\tFF\tFF\tFF\tFF\tFF\tFF\r\n      3952  1FFFFFFF   00000004    8        00\t00\tFF\tFF\tFF\tFF\tFF\tFF\r\n      3947  1FFFFFFF   00000004    8        00\t00\tFF\tFF\tFF\tFF\tFF\tFF\r\n      3946  18F121F0   00000004    8        09\t33\t00\t00\tFF\tFF\tB0\t01\r\n      3945  18F106A7   00000004    8        00\tF7\tFF\tFF\tFF\tFF\tFF\tBF\r\n      3945  0CF104A7   00000004    8        F0\t60\t22\tFC\tFF\tFF\tFF\t5F\r\n      3944  0CF103A7   00000004    8        17\t1F\t08\t60\tB1\t1F\t08\t5F\r\n      3944  0CF102A7   00000004    8        30\t75\tE0\t2E\t80\tFF\tFF\tFD\r\n      3943  0C3C4D4A   00000004    8        BE\tFF\tFF\t7F\t18\tFF\tFF\t5F\r\n      3972  1FFFFFFF   00000004    8        00\t00\tFF\tFF\tFF\tFF\tFF\tFF\r\n      3963  0CF102A7   00000004    8        30\t75\tE0\t2E\t80\tFF\tFF\tFD\r\n      3963  0CF101A7   00000004    8        68\t00\t97\tCC\t00\t19\t39\tE0\r\n      3962  1FFFFFFF   00000004    8        00\t00\tFF\tFF\tFF\tFF\tFF\tFF\r\n      3952  1FFFFFFF   00000004    8        00\t00\tFF\tFF\tFF\tFF\tFF\tFF\r\n      3947  1FFFFFFF   00000004    8        00\t00\tFF\tFF\tFF\tFF\tFF\tFF\r\n      3946  18F121F0   00000004    8        09\t33\t00\t00\tFF\tFF\tB0\t01\r\n      3945  18F106A7   00000004    8        00\tF7\tFF\tFF\tFF\tFF\tFF\tBF\r\n      3945  0CF104A7   00000004    8        F0\t60\t22\tFC\tFF\tFF\tFF\t5F\r\n      3944  0CF103A7   00000004    8        17\t1F\t08\t60\tB1\t1F\t08\t5F\r\n      3944  0CF102A7   00000004    8        30\t75\tE0\t2E\t80\tFF\tFF\tFD\r\n      3982  1FFFFFFF   00000004    8        00\t00\tFF\tFF\tFF\tFF\tFF\tFF\r\n      3972  1FFFFFFF   00000004    8        00\t00\tFF\tFF\tFF\tFF\tFF\tFF\r\n      3963  0CF102A7   00000004    8        30\t75\tE0\t2E\t80\tFF\tFF\tFD\r\n      3963  0CF101A7   00000004    8        68\t00\t97\tCC\t00\t19\t39\tE0\r\n      3962  1FFFFFFF   00000004    8        00\t00\tFF\tFF\tFF\tFF\tFF\tFF\r\n      3952  1FFFFFFF   00000004    8        00\t00\tFF\tFF\tFF\tFF\tFF\tFF\r\n      3947  1FFFFFFF   00000004    8        00\t00\tFF\tFF\tFF\tFF\tFF\tFF\r\n      3946  18F121F0   00000004    8        09\t33\t00\t00\tFF\tFF\tB0\t01\r\n      3945  18F106A7   00000004    8        00\tF7\tFF\tFF\tFF\tFF\tFF\tBF\r\n      3945  0CF104A7   00000004    8        F0\t60\t22\tFC\tFF\tFF\tFF\t5F\r\n      3944  0CF103A7   00000004    8        17\t1F\t08\t60\tB1\t1F\t08\t5F\r\n      3983  0CF101A7   00000004    8        68\t00\t97\tCC\t00\t19\t39\tE1\r\n      3982  1FFFFFFF   00000004    8        00\t00\tFF\tFF\tFF\tFF\tFF\tFF\r\n      3972  1FFFFFFF   00000004    8        00\t00\tFF\tFF\tFF\tFF\tFF\tFF\r\n      3963  0CF102A7   00000004    8        30\t75\tE0\t2E\t80\tFF\tFF\tFD\r\n      3963  0CF101A7   00000004    8        68\t00\t97\tCC\t00\t19\t39\tE0\r\n      3962  1FFFFFFF   00000004    8        00\t00\tFF\tFF\tFF\tFF\tFF\tFF\r\n      3952  1FFFFFFF   00000004    8        00\t00\tFF\tFF\tFF\tFF\tFF\tFF\r\n      3947  1FFFFFFF   00000004    8        00\t00\tFF\tFF\tFF\tFF\tFF\tFF\r\n      3946  18F121F0   00000004    8        09\t33\t00\t00\tFF\tFF\tB0\t01\r\n      3945  18F106A7   00000004    8        00\tF7\tFF\tFF\tFF\tFF\tFF\tBF\r\n      3945  0CF104A7   00000004    8        F0\t60\t22\tFC\tFF\tFF\tFF\t5F\r\n      3983  0CF102A7   00000004    8        30\t75\tE0\t2E\t80\tFF\tFF\tFD\r\n      3983  0CF101A7   00000004    8        68\t00\t97\tCC\t00\t19\t39\tE1\r\n      3982  1FFFFFFF   00000004    8        00\t00\tFF\tFF\tFF\tFF\tFF\tFF\r\n      3972  1FFFFFFF   00000004    8        00\t00\tFF\tFF\tFF\tFF\tFF\tFF\r\n      3963  0CF102A7   00000004    8        30\t75\tE0\t2E\t80\tFF\tFF\tFD\r\n      3963  0CF101A7   00000004    8        68\t00\t97\tCC\t00\t19\t39\tE0\r\n      3962  1FFFFFFF   00000004    8        00\t00\tFF\tFF\tFF\tFF\tFF\tFF\r\n      3952  1FFFFFFF   00000004    8        00\t00\tFF\tFF\tFF\tFF\tFF\tFF\r\n      3947  1FFFFFFF   00000004    8        00\t00\tFF\tFF\tFF\tFF\tFF\tFF\r\n      3946  18F121F0   00000004    8        09\t33\t00\t00\tFF\tFF\tB0\t01\r\n      3945  18F106A7   00000004    8        00\tF7\tFF\tFF\tFF\tFF\tFF\tBF\r\n      3992  1FFFFFFF   00000004    8        00\t00\tFF\tFF\tFF\tFF\tFF\tFF\r\n      3983  0CF102A7   00000004    8        30\t75\tE0\t2E\t80\tFF\tFF\tFD\r\n      3983  0CF101A7   00000004    8        68\t00\t97\tCC\t00\t19\t39\tE1\r\n      3982  1FFFFFFF   00000004    8        00\t00\tFF\tFF\tFF\tFF\tFF\tFF\r\n      3972  1FFFFFFF   00000004    8        00\t00\tFF\tFF\tFF\tFF\tFF\tFF\r\n      3963  0CF102A7   00000004    8        30\t75\tE0\t2E\t80\tFF\tFF\tFD\r\n      3963  0CF101A7   00000004    8        68\t00\t97\tCC\t00\t19\t39\tE0\r\n      3962  1FFFFFFF   00000004    8        00\t00\tFF\tFF\tFF\tFF\tFF\tFF\r\n      3952  1FFFFFFF   00000004    8        00\t00\tFF\tFF\tFF\tFF\tFF\tFF\r\n      3947  1FFFFFFF   00000004    8        00\t00\tFF\tFF\tFF\tFF\tFF\tFF\r\n      3946  18F121F0   00000004    8        09\t33\t00\t00\tFF\tFF\tB0\t01\r\n      3993  18F106A7   00000004    8        00\tF7\tFF\tFF\tFF\tFF\tFF\tC0\r\n      3992  1FFFFFFF   00000004    8        00\t00\tFF\tFF\tFF\tFF\tFF\tFF\r\n      3983  0CF102A7   00000004    8        30\t75\tE0\t2E\t80\tFF\tFF\tFD\r\n      3983  0CF101A7   00000004    8        68\t00\t97\tCC\t00\t19\t39\tE1\r\n      3982  1FFFFFFF   00000004    8        00\t00\tFF\tFF\tFF\tFF\tFF\tFF\r\n      3972  1FFFFFFF   00000004    8        00\t00\tFF\tFF\tFF\tFF\tFF\tFF\r\n      3963  0CF102A7   00000004    8        30\t75\tE0\t2E\t80\tFF\tFF\tFD\r\n      3963  0CF101A7   00000004    8        68\t00\t97\tCC\t00\t19\t39\tE0\r\n      3962  1FFFFFFF   00000004    8        00\t00\tFF\tFF\tFF\tFF\tFF\tFF\r\n      3952  1FFFFFFF   00000004    8        00\t00\tFF\tFF\tFF\tFF\tFF\tFF\r\n      3947  1FFFFFFF   00000004    8        00\t00\tFF\tFF\tFF\tFF\tFF\tFF\r\n      4002  1FFFFFFF   00000004    8        00\t00\tFF\tFF\tFF\tFF\tFF\tFF\r\n      3993  18F106A7   00000004    8        00\tF7\tFF\tFF\tFF\tFF\tFF\tC0\r\n      3992  1FFFFFFF   00000004    8        00\t00\tFF\tFF\tFF\tFF\tFF\tFF\r\n      3983  0CF102A7   00000004    8        30\t75\tE0\t2E\t80\tFF\tFF\tFD\r\n      3983  0CF101A7   00000004    8        68\t00\t97\tCC\t00\t19\t39\tE1\r\n      3982  1FFFFFFF   00000004    8        00\t00\tFF\tFF\tFF\tFF\tFF\tFF\r\n      3972  1FFFFFFF   00000004    8        00\t00\tFF\tFF\tFF\tFF\tFF\tFF\r\n      3963  0CF102A7   00000004    8        30\t75\tE0\t2E\t80\tFF\tFF\tFD\r\n      3963  0CF101A7   00000004    8        68\t00\t97\tCC\t00\t19\t39\tE0\r\n      3962  1FFFFFFF   00000004    8        00\t00\tFF\tFF\tFF\tFF\tFF\tFF\r\n      3952  1FFFFFFF   00000004    8        00\t00\tFF\tFF\tFF\tFF\tFF\tFF\r\n      4002  0CF101A7   00000004    8        68\t00\t97\tCC\t00\t19\t39\tE2\r\n      4002  1FFFFFFF   00000004    8        00\t00\tFF\tFF\tFF\tFF\tFF\tFF\r\n      3993  18F106A7   00000004    8        00\tF7\tFF\tFF\tFF\tFF\tFF\tC0\r\n      3992  1FFFFFFF   00000004    8        00\t00\tFF\tFF\tFF\tFF\tFF\tFF\r\n      3983  0CF102A7   00000004    8        30\t75\tE0\t2E\t80\tFF\tFF\tFD\r\n      3983  0CF101A7   00000004    8        68\t00\t97\tCC\t00\t19\t39\tE1\r\n      3982  1FFFFFFF   00000004    8        00\t00\tFF\tFF\tFF\tFF\tFF\tFF\r\n      3972  1FFFFFFF   00000004    8        00\t00\tFF\tFF\tFF\tFF\tFF\tFF\r\n      3963  0CF102A7   00000004    8        30\t75\tE0\t2E\t80\tFF\tFF\tFD\r\n      3963  0CF101A7   00000004    8        68\t00\t97\tCC\t00\t19\t39\tE0\r\n      3962  1FFFFFFF   00000004    8        00\t00\tFF\tFF\tFF\tFF\tFF\tFF\r\n      4003  0CF102A7   00000004    8        30\t75\tE0\t2E\t80\tFF\tFF\tFD\r\n      4002  0CF101A7   00000004    8        68\t00\t97\tCC\t00\t19\t39\tE2\r\n      4002  1FFFFFFF   00000004    8        00\t00\tFF\tFF\tFF\tFF\tFF\tFF\r\n      3993  18F106A7   00000004    8        00\tF7\tFF\tFF\tFF\tFF\tFF\tC0\r\n      3992  1FFFFFFF   00000004    8        00\t00\tFF\tFF\tFF\tFF\tFF\tFF\r\n      3983  0CF102A7   00000004    8        30\t75\tE0\t2E\t80\tFF\tFF\tFD\r\n      3983  0CF101A7   00000004    8        68\t00\t97\tCC\t00\t19\t39\tE1\r\n      3982  1FFFFFFF   00000004    8        00\t00\tFF\tFF\tFF\tFF\tFF\tFF\r\n      3972  1FFFFFFF   00000004    8        00\t00\tFF\tFF\tFF\tFF\tFF\tFF\r\n      3963  0CF102A7   00000004    8        30\t75\tE0\t2E\t80\tFF\tFF\tFD\r\n      3963  0CF101A7   00000004    8        68\t00\t97\tCC\t00\t19\t39\tE0\r\n      4012  1FFFFFFF   00000004    8        00\t20\tFF\tFF\tFF\tFF\tFF\tFF\r\n      4003  0CF102A7   00000004    8        30\t75\tE0\t2E\t80\tFF
